vi "DoubleArray_To_NumpyArrayString.vi"(4 "double array":dbl[](array[numeric])) -> (1 "data string":string, 2 "descriptor":string)   [LabVIEW 2016, in "PyLVi.lvlib" / "PyLVi.lvclass"]
uses:
  PyLVi.lvclass
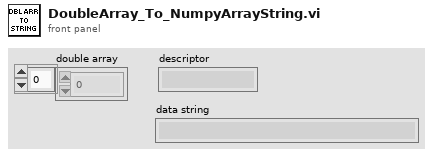
[diagram p1: front panel]
types:
  T1 = enum16{"big-endian, network order", "native, host order", "little-endian"}
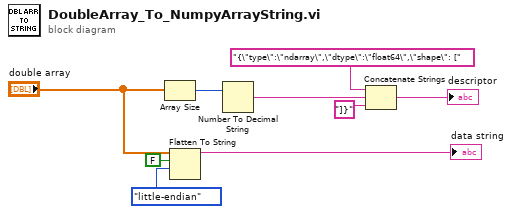
[diagram p0: block diagram]
diagram:
  n1 = Array Size(array="double array") -> (size(s)=w7:i32)
  n2 = Flatten To String(anything="double array", prepend array or string size? (T)=FALSE, byte order (0:big-endian, network order)=T1."little-endian") -> (data string=→"data string":string)  [unwired: 1 in, 2 out]
  n3 = Number To Decimal String(number=w7) -> (decimal integer string=w6:string)  [unwired: 1 in]
  n4 = Concatenate Strings("{\"type\":\"ndarray\",\"dtype\":\"float64\",\"shape\": [" ("string"), w6, "]}" ("string")) -> (→"descriptor":string)
